vi "PulseModEntry.vi"(0 "OnTimeSet":bool, 1 "Keypad In":dbl, 5 "OnT ini":u16=1, 7 "OffTimeSet":bool, 9 "OffT ini":u16=15, 11 "PulsesSet":bool, 12 "Pulses ini":u32=65535, 13 "OffpwrSet":bool, 14 "Off Pwr ini":u8=64) -> (3 "reset":bool, 4 "OnTime":u16=1, 8 "OffTime":u16=15, 10 "NumPulses":u32=65535, 15 "Off Power":u8=255)   [LabVIEW 2012]
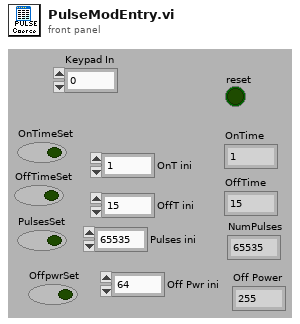
[diagram p1: front panel]
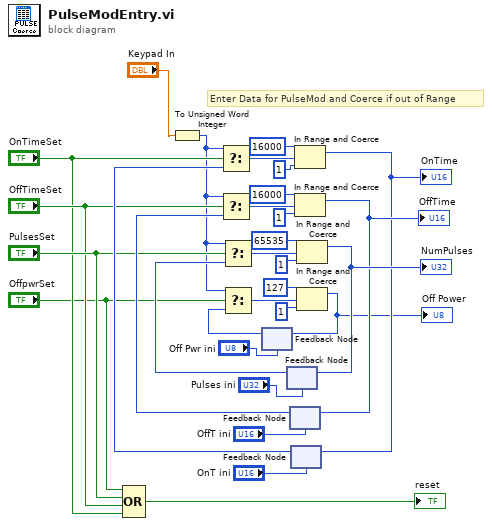
[diagram p0: block diagram]
diagram:
  # "Enter Data for PulseMod and Coerce if out of Range"
  n1 = Compound Arithmetic op=OR("OffpwrSet", "PulsesSet", "OffTimeSet", "OnTimeSet") -> (→"reset":bool)
  n2 = To Unsigned Word Integer(number="Keypad In") -> (unsigned 16bit integer=w3:u16)
  n3 = feedback #1("Off Pwr ini") -> (w5:u32)
  n4 = Select(t=w3, s="OffpwrSet", f=w5) -> (s? t:f=w7:u32)
  n5 = feedback #2("Pulses ini") -> (w24:u32)
  n6 = Select(t=w3, s="PulsesSet", f=w24) -> (s? t:f=w27:u32)
  n7 = feedback #3("OffT ini") -> (w21:u16)
  n8 = Select(t=w3, s="OffTimeSet", f=w21) -> (s? t:f=w29:u16)
  n9 = feedback #4("OnT ini") -> (w16:u16)
  n10 = Select(t=w3, s="OnTimeSet", f=w16) -> (s? t:f=w18:u16)
  n11 = In Range and Coerce(upper limit=u16 16000, x=w18, lower limit=u16 1) -> (coerced(x)=w17:u16)  [unwired: 1 out]
  "OnTime" <- w17
  n12 = feedback-in #4(w17) -> ()
  n13 = In Range and Coerce(upper limit=u16 16000, x=w29, lower limit=u16 1) -> (coerced(x)=w22:u16)  [unwired: 1 out]
  "OffTime" <- w22
  n14 = feedback-in #3(w22) -> ()
  n15 = In Range and Coerce(upper limit=u32 65535, x=w27, lower limit=u32 1) -> (coerced(x)=w25:u32)  [unwired: 1 out]
  "NumPulses" <- w25
  n16 = feedback-in #2(w25) -> ()
  n17 = In Range and Coerce(upper limit=u32 127, x=w7, lower limit=u32 1) -> (coerced(x)=w1:u32)  [unwired: 1 out]
  "Off Power" <- w1
  n18 = feedback-in #1(w1) -> ()
